vi "Send to Caller.vi"(8 "error in (no error)":errorcluster, 9 "Priority (Normal)":T1=enum."Normal", 10 "Message":refnum<class "Message.lvclass">, 11 "Actor in":refnum<class "Actor.lvclass">) -> (0 "error out":errorcluster, 3 "Actor out":refnum<class "Actor.lvclass">)   [LabVIEW 2020, in "Artifex.lvlib" / "Actor.lvclass"]
uses:
  Actor.lvclass
  Actor Proxy/Actor API.lvclass
  Message/Message.lvclass
  Priority.ctl
  Artifex.lvlib
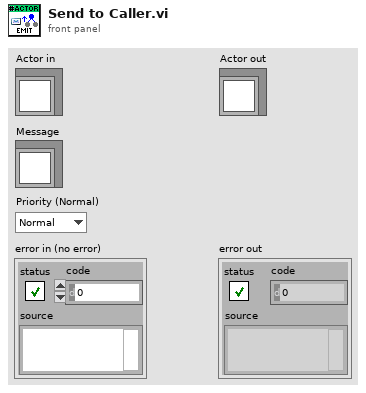
[diagram p1: front panel]
types:
  T1 = typedef "Artifex.lvlib/Priority.ctl" = enum16{"Low", "Normal", "High"}
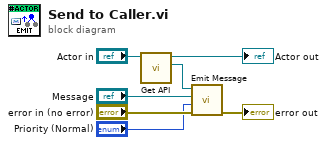
[diagram p0: block diagram]
diagram:
  n1 = call-dynamic "Get API.vi"("Actor in"="Actor in") -> ("Actor API"=w2:refnum<class "Actor API.lvclass">, "Actor out"=→"Actor out":refnum<class "Actor.lvclass">)  [unwired: 8 in, 1 out]
  n2 = call "Emit Message.vi"("error in (no error)"="error in (no error)", "Priority (Normal)"="Priority (Normal)", "Message"="Message", "Actor API in"=w2) -> ("error out"=→"error out":errorcluster)  [unwired: 6 in, 1 out]
